vi "Timer.vi"(7 "Timer CMD":T1, 8 "error in (no error)":errorcluster, 11 "Target Time":dbl) -> (0 "error out":errorcluster, 2 "Elapsed?":bool, 3 "Elapsed Time":dbl)   [LabVIEW 2017]
doc: "Timer based on Functional Global Variable."
uses:
  Controls/Timer CMD.ctl
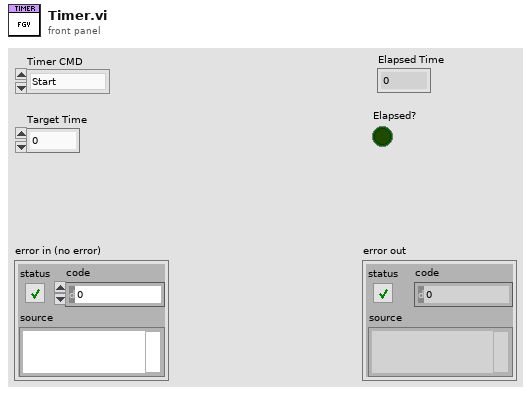
[diagram p1: front panel]
types:
  T1 = typedef "Timer CMD.ctl" = enum16{"Start", "Restart", "Get Time", "Pause", "UnPause"}
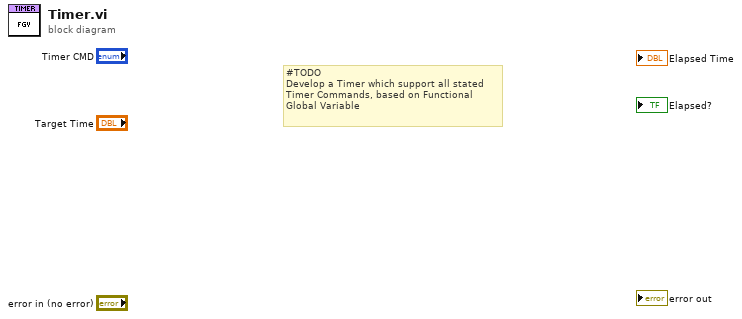
[diagram p0: block diagram]
diagram:
  # "#TODO\nDevelop a Timer which support all stated\nTimer Commands, based on Functional\nGlobal Variable"
